vi "Example One Stage.vi"() -> ()   [LabVIEW 2019]
uses:
  Class/Controller/Controller.lvclass
  <vilib>/Platform/TimedLoop/XDataNode/timing_clust.ctl
  <vilib>/Platform/TimedLoop/XDataNode/nitl_modes.ctl
  <vilib>/Platform/TimedLoop/XDataNode/wakeup.ctl
  <vilib>/platform/TimedLoop/XDataNode/XDataNode.xnode
  <vilib>/Platform/TimedLoop/XDataNode/XDNodeRunTimeDep.lvlib
panel:
  out "Desired Position\n[selected units]":dbl
  out "Encoder position \n[selected units]":dbl
  in  "Tab Control":enum32{"Motion", "Settings"}(tab)
  in  "Zero Output":bool
  in  "Go to Home":bool
  in  "Scan Right":bool
  in  "Scan Left":bool
  in  "Continue":bool
  in  "Stop":bool
  in  "Make Step Right":bool
  in  "Step Size \n[selected units]":dbl=1.0 format="%#.2f"
  in  "Make Step Left":bool
  in  "Desired Speed \n[1µm/s or 0,01deg /s]":dbl=10000.0 format="%#.2f"
  in  "Desired Position \n[selected units]":dbl format="%#.2f"
  in  "Find Index":bool
  in  "Reset":bool
  out "error out":errorcluster
  in  "Working Units":string(combo)="1000000"
  out "StatusBits":T1
  out "Status Info":T2
  in  "Axis Resolution":string(combo)="312.5"
  in  "Axis Letter":string="X"
  in  "Baudrate":dbl=9600.0
  in  "COM Port":refnum<visa-resource-name>
  in  "Controller.lvclass":refnum<class "Controller.lvclass">
  out "Waveform Chart":dbl(graph)=-0.078
  in  "STOP PROGRAM":bool
  # "Visualization"
  # "Extra information"
  # "READ ME FIRST"
  # "Configuration"
  # "Stage 1"
  # "Driver 1"
  # "Stage 1"
  # "How to run:"
  # "BEFORE RUNNING:"
  # "1, Select COM Port"
  # "2. Select baudrate"
  # "3. For each axis:"
  # "3.1 Specify correct axis name (1 letter)"
  # "3.2 Specify correct resolution"
  # "4. Run VI"
  # "WHEN RUNNING, YOU HAVE TO FIRST PUSH \"FIND INDEX\" FOR EACH STAGE.\nThe stages will start moving and find its position. After that you can control the stages"
  # "NOTES: Do this only the first time"
  # "1. Replace the settings_default.txt file with\nthe file we provided on a USB stick."
  # "2.    Make sure there are no comments in the\nsettings_default.txt file. ONLY lines like: \"X:DPOS=100\" so NO \"%\" in front or at the end of the line."
  # "Position Information"
  # "STOP BUTTON"
  # "3.  In your settings_default.txt file:\nEvery line that contains SSPD or MSPD: multiply that value with:\n - 1000 for a lineair stage \n - 100 for a rotating stage"
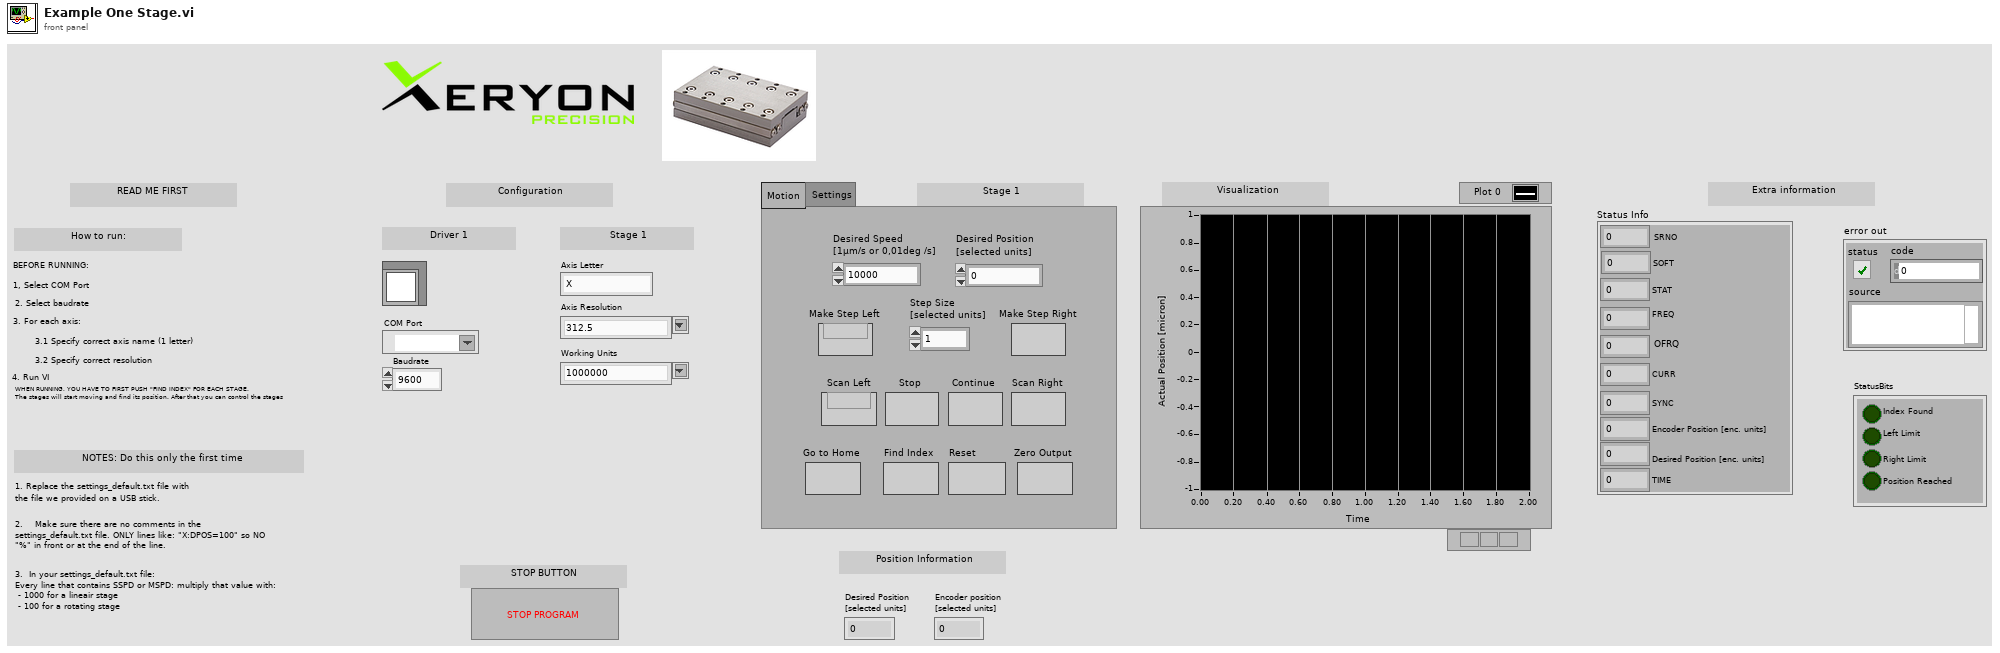
[diagram p1: front panel]
types:
  T1 = cluster{"Index Found":bool, "Left Limit":bool, "Right Limit":bool, "Position Reached":bool}
  T2 = cluster{"SRNO":dbl, "SOFT":dbl, "STAT":dbl, "FREQ":dbl, "OFRQ":dbl, "CURR":dbl, "SYNC":dbl, "Encoder Position [enc. units]":dbl, "Desired Position [enc. units]":dbl, "TIME":dbl}
  T3 = typedef "XDNodeRunTimeDep.lvlib/timing_clust.ctl" = cluster{"Expected End [f-1]":u64, "Actual End [f-1]":u64, "Finished Late? [f-1]":bool, "Expected End [i-1]":u64, "Actual End [i-1]":u64, "Finished Late? [i-1]":bool, "Expected Start [i]":u64, "Actual Start [i]":u64, "Expected Start [f]":u64, "Actual Start [f]":u64, "Source Name":string, "Structure Name":string, "Period":i64, "Deadline":i64, "Offset":i64, "Start":i64, "Priority":i32, "Timeout":i32, "Mode":T4, "Wakeup Reason":T5, "Error":errorcluster, "Source Type":string, "Secondary Source Type":string, "Global End Time":u64, "Global Start Time":u64, "Frame Duration":u64, "Iteration Duration":u64, "Assigned CPU":i32, "I/O Scan Engine Mode":u32}
  T4 = typedef "XDNodeRunTimeDep.lvlib/nitl_modes.ctl" = enum32{"No Change", "Process missed periods, maintain original phase", "Discard missed periods, maintain original phase", "Process missed periods, ignore original phase", "Discard missed periods, ignore original phase"}
  T5 = typedef "XDNodeRunTimeDep.lvlib/wakeup.ctl" = enum32{"Normal", "Aborted", "Asynchronous wakeup", "Timing source error", "Timed loop error", "Timeout"}
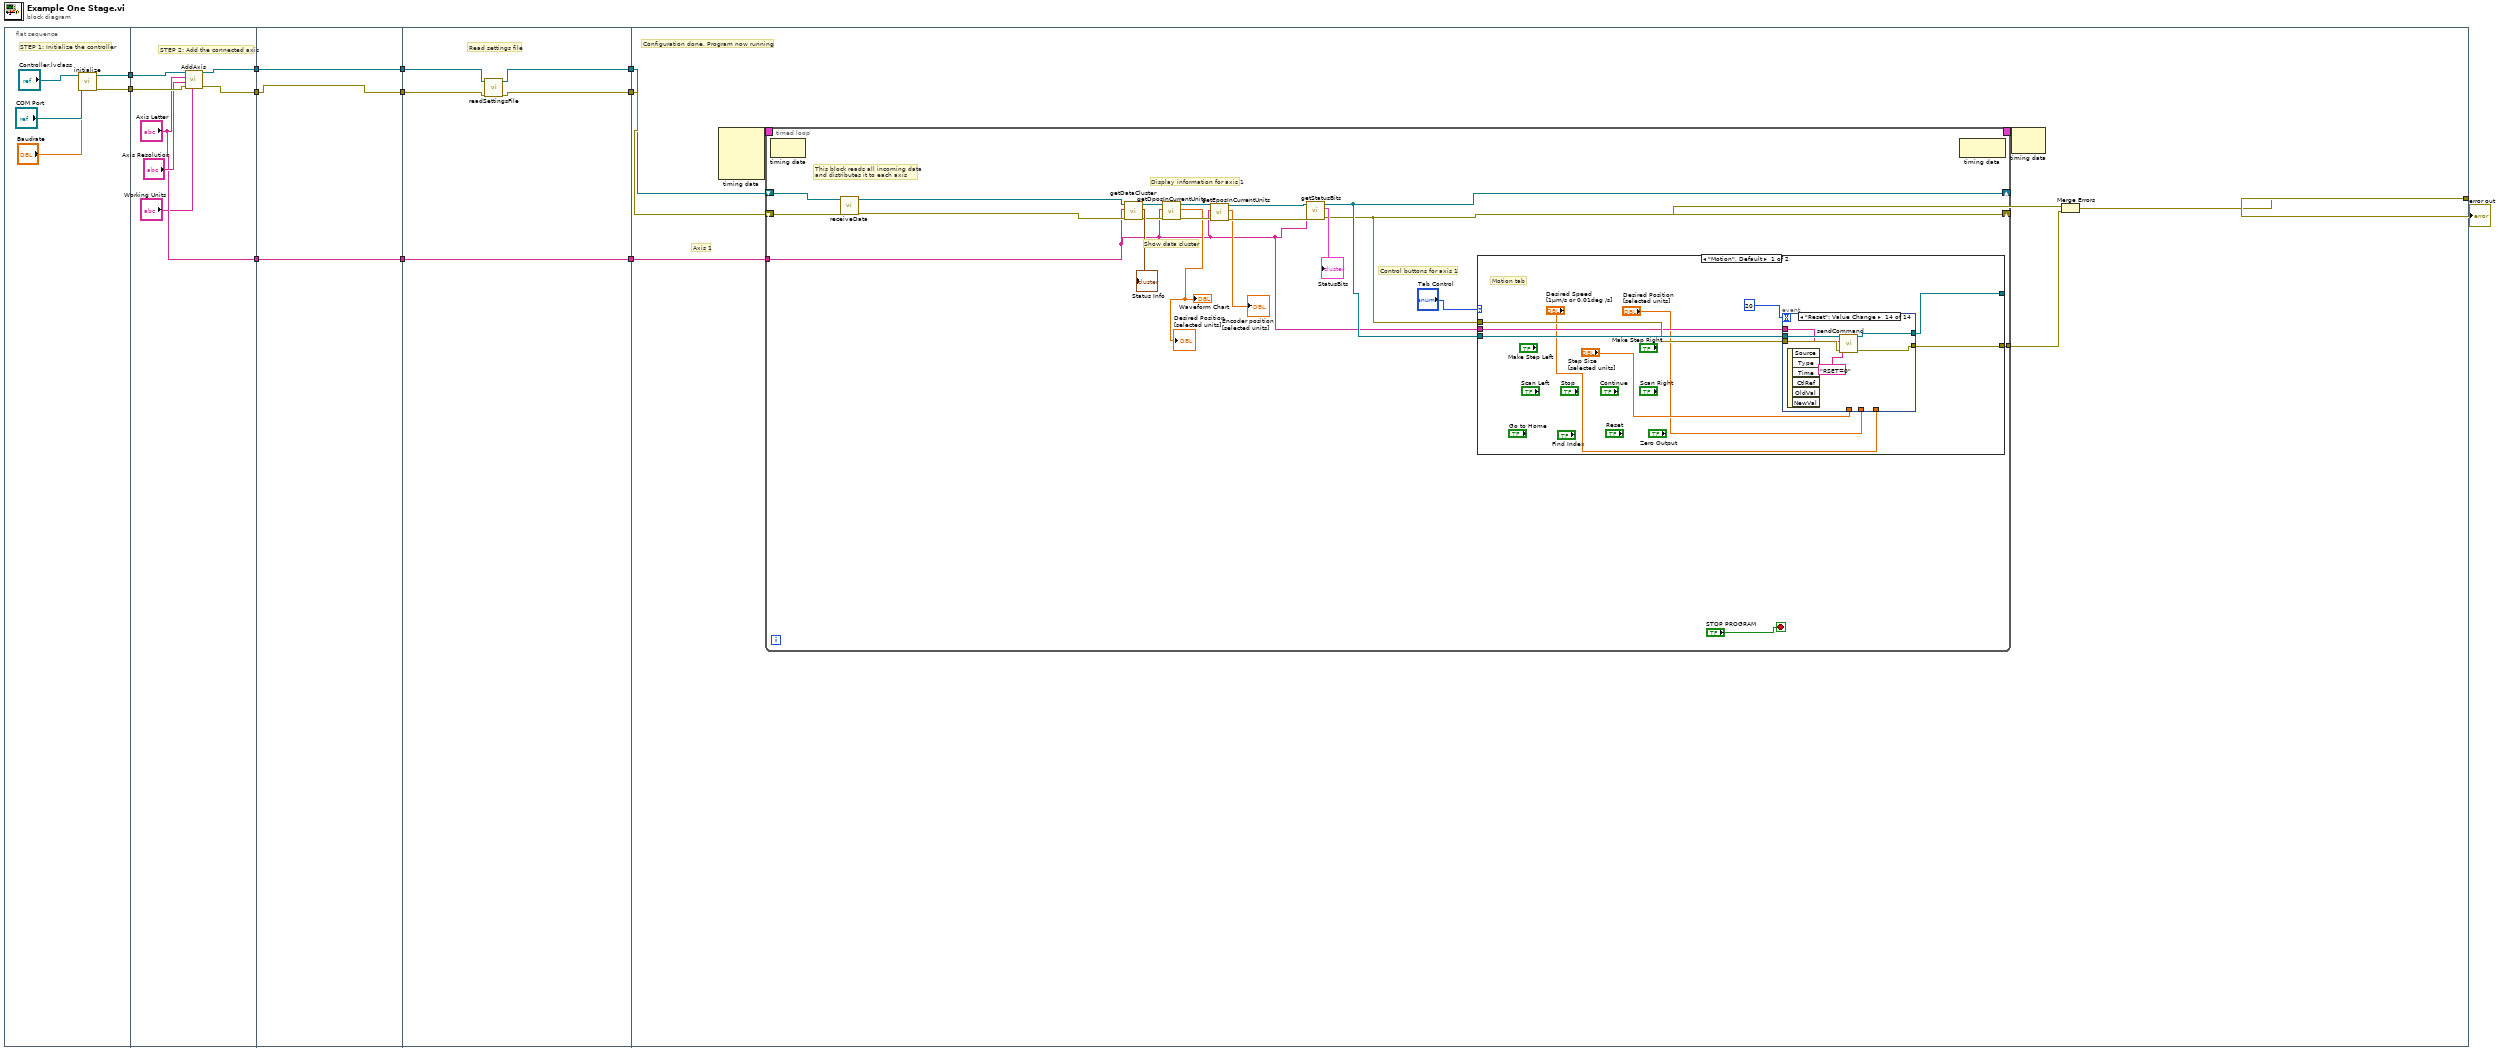
[diagram p0: block diagram]
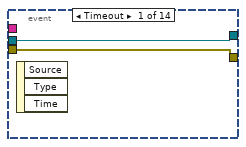
[diagram p2: hidden frame]
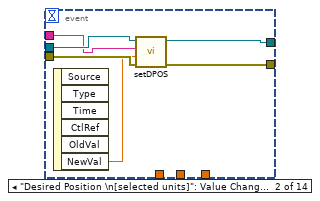
[diagram p3: hidden frame]
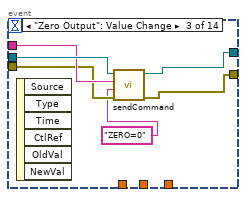
[diagram p4: hidden frame]
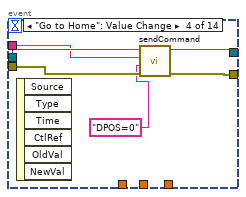
[diagram p5: hidden frame]
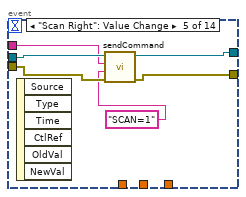
[diagram p6: hidden frame]
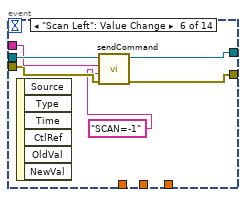
[diagram p7: hidden frame]
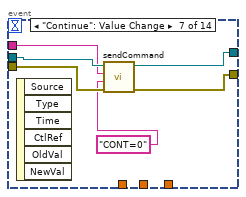
[diagram p8: hidden frame]
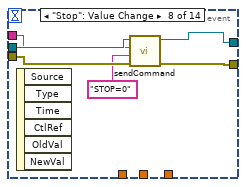
[diagram p9: hidden frame]
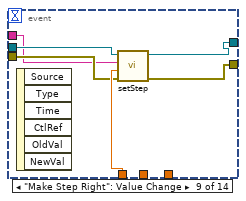
[diagram p10: hidden frame]
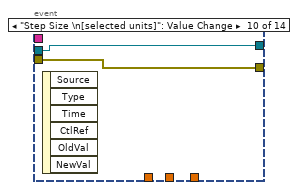
[diagram p11: hidden frame]
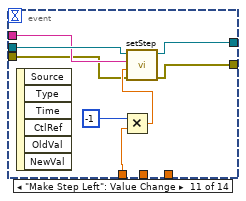
[diagram p12: hidden frame]
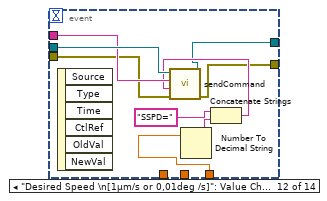
[diagram p13: hidden frame]
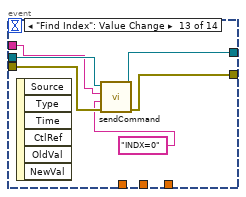
[diagram p14: hidden frame]
diagram:
  n1 = flat-sequence {
    tunnel: [w14] -> w12
    tunnel: [w13] -> w11
    tunnel: w12 -> [w24]
    tunnel: w11 -> [w23]
    tunnel: [w21] -> w10
    tunnel: [w20] -> w9
    tunnel: ["Axis Letter"] -> w8
    tunnel: w10 -> [w26]
    tunnel: w9 -> [w25]
    tunnel: [w27] -> w6
    tunnel: w8 -> [w27]
    tunnel: [w26] -> w4
    tunnel: [w25] -> w2
    tunnel: w6 -> [w32]
    tunnel: [w32] -> w5
    tunnel: w4 -> [w31]
    tunnel: [w29] -> w3
    tunnel: w2 -> [w30]
    tunnel: [w28] -> w1
    tunnel: w5 -> [w33]
    tunnel: w3 -> [w39]
    tunnel: w1 -> [w40]
    tunnel: [w35] -> w7
    frame #0 {
      # "STEP 1: Initialize the controller"
      n2 = call-dynamic "initialize.vi"("Baudrate"="Baudrate", "COM Port"="COM Port", "Controller in"="Controller.lvclass") -> ("error out"=w13:errorcluster, "Controller out"=w14:refnum<class "Controller.lvclass">)  [unwired: 7 in]
    }
    frame #1 {
      # "STEP 2: Add the connected axis"
      n3 = call-dynamic "AddAxis.vi"("Units"="Working Units", "error in (no error)"=w23, "Encoder Resolution"="Axis Resolution", "Axis Letter"="Axis Letter", "Controller in"=w24) -> ("error out"=w20:errorcluster, "Controller out"=w21:refnum<class "Controller.lvclass">)  [unwired: 5 in]
    }
    frame #2 {
    }
    frame #3 {
      # "Read settings file"
      n4 = call-dynamic "readSettingsFile.vi"("error in (no error)"=w30, "Controller in"=w31) -> ("error out"=w28:errorcluster, "Controller out"=w29:refnum<class "Controller.lvclass">)  [unwired: 8 in]
    }
    frame #4 {
      # "Axis 1"
      # "Configuration done. Program now running"
      n5 = node-c288() -> (w38:T3)  [unwired: 4 in]
      n6 = timed-loop {
        shift-right: [w44] -> _
        shift-left: w39 -> [w60]
        tunnel: w33 -> [w42]
        shift-right: [w43] -> w36
        shift-left: w40 -> [w47]
        timing: w38 -> [_]
        timing-out: [_] -> w37
        tunnel: [w41] -> w34
        stop <- "STOP PROGRAM" stop-if-true
        # "Control buttons for axis 1"
        # "Display information for axis 1"
        # "Show data cluster"
        # "This block reads all incoming data\nand distributes it to each axis"
        n7 = node-c288() -> ()  [unwired: 1 in, 1 out]
        n8 = call-dynamic "receiveData.vi"("error in (no error)"=w47, "Controller in"=w60) -> ("error out"=w58:errorcluster, "Controller out"=w59:refnum<class "Controller.lvclass">)  [unwired: 8 in]
        n9 = call-dynamic "getDataCluster.vi"("error in (no error)"=w58, "Axis Letter"=w42, "Controller in"=w59) -> ("error out"=w52:errorcluster, "Information"=→"Status Info":T2, "Controller out"=w55:refnum<class "Controller.lvclass">)  [unwired: 6 in]
        n10 = call-dynamic "getDposInCurrentUnits.vi"("error in (no error)"=w52, "Axis Letter"=w42, "Controller in"=w55) -> ("error out"=w51:errorcluster, "DPOS In Current Units"=→"Waveform Chart" →"Desired Position\n[selected units]":dbl, "Controller out"=w54:refnum<class "Controller.lvclass">)  [unwired: 6 in]
        n11 = call-dynamic "getEposInCurrentUnits.vi"("error in (no error)"=w51, "Axis Letter"=w42, "Controller in"=w54) -> ("error out"=w50:errorcluster, "EPOS In Current Units"=→"Encoder position \n[selected units]":dbl, "Controller out"=w53:refnum<class "Controller.lvclass">)  [unwired: 6 in]
        n12 = call-dynamic "getStatusBits.vi"("error in (no error)"=w50, "Axis Letter"=w42, "Controller in"=w53) -> ("error out"=w43:errorcluster, "StatusBits"=→"StatusBits":T1, "Controller out"=w44:refnum<class "Controller.lvclass">)  [unwired: 6 in]
        n13 = case shown="\"Motion\", Default" "Tab Control" {
          tunnel: w44 -> [w69 w151]
          tunnel: w43 -> [w68 w152]
          tunnel: [w67 w151] -> _
          tunnel: [w66 w152] -> w41
          tunnel: w42 -> [w64 _]
          frame "Motion", Default {
            # "Motion tab"
            n14 = event shown="[13] \"Reset\": Value Change" {
              selector: _ -> [_ _ _ _ _ _ _ _ _ _ _ _ _ _]
              dyn-events: _ -> [_ _ _ _ _ _ _ _ _ _ _ _ _ _]
              timeout: 20 -> [_ _ _ _ _ _ _ _ _ _ _ _ _ _]
              tunnel: w69 -> [w71 w77 w83 w89 w95 w101 w107 w113 w117 w121 w127 w138 w144 w150]
              tunnel: w68 -> [w70 w76 w81 w87 w93 w99 w105 w111 w118 w120 w124 w136 w142 w149]
              tunnel: [w71 w74 w79 w84 w91 w97 w103 w109 w115 w121 w122 w130 w140 w146] -> w67
              tunnel: [w70 w75 w80 w86 w92 w98 w104 w110 w114 w120 w123 w131 w141 w145] -> w66
              tunnel: w64 -> [_ w72 w82 w88 w94 w100 w106 w112 w116 _ w126 w137 w143 w148]
              tunnel: "Step Size \n[selected units]" -> [_ _ _ _ _ _ _ _ w119 _ w128 _ _ _]
              tunnel: "Desired Position \n[selected units]" -> [_ _ _ _ _ _ _ _ _ _ _ _ _ _]
              tunnel: "Desired Speed \n[1µm/s or 0,01deg /s]" -> [_ _ _ _ _ _ _ _ _ _ _ w135 _ _]
              event Timeout {
                n15 = event-data() -> ()  [unwired: 1 in, 3 out]
              }
              event "Desired Position \n[selected units]": Value Change {
                n16 = event-data() -> ("NewVal"=w73:dbl)  [unwired: 1 in, 5 out]
                n17 = call-dynamic "setDPOS.vi"("error in (no error)"=w76, "DPOS In Current Units"=w73, "Axis Letter"=w72, "Controller in"=w77) -> ("error out"=w75:errorcluster, "Controller out"=w74:refnum<class "Controller.lvclass">)  [unwired: 6 in]
              }
              event "Zero Output": Value Change {
                n18 = event-data() -> ()  [unwired: 1 in, 6 out]
                n19 = call-dynamic "sendCommand.vi"("error in (no error)"=w81, "Command"="ZERO=0", "Axis Letter"=w82, "Controller in"=w83) -> ("error out"=w80:errorcluster, "Controller out"=w79:refnum<class "Controller.lvclass">)  [unwired: 6 in]
              }
              event "Go to Home": Value Change {
                n20 = event-data() -> ()  [unwired: 1 in, 6 out]
                n21 = call-dynamic "sendCommand.vi"("error in (no error)"=w87, "Command"="DPOS=0", "Axis Letter"=w88, "Controller in"=w89) -> ("error out"=w86:errorcluster, "Controller out"=w84:refnum<class "Controller.lvclass">)  [unwired: 6 in]
              }
              event "Scan Right": Value Change {
                n22 = event-data() -> ()  [unwired: 1 in, 6 out]
                n23 = call-dynamic "sendCommand.vi"("error in (no error)"=w93, "Command"="SCAN=1", "Axis Letter"=w94, "Controller in"=w95) -> ("error out"=w92:errorcluster, "Controller out"=w91:refnum<class "Controller.lvclass">)  [unwired: 6 in]
              }
              event "Scan Left": Value Change {
                n24 = event-data() -> ()  [unwired: 1 in, 6 out]
                n25 = call-dynamic "sendCommand.vi"("error in (no error)"=w99, "Command"="SCAN=-1", "Axis Letter"=w100, "Controller in"=w101) -> ("error out"=w98:errorcluster, "Controller out"=w97:refnum<class "Controller.lvclass">)  [unwired: 6 in]
              }
              event "Continue": Value Change {
                n26 = event-data() -> ()  [unwired: 1 in, 6 out]
                n27 = call-dynamic "sendCommand.vi"("error in (no error)"=w105, "Command"="CONT=0", "Axis Letter"=w106, "Controller in"=w107) -> ("error out"=w104:errorcluster, "Controller out"=w103:refnum<class "Controller.lvclass">)  [unwired: 6 in]
              }
              event "Stop": Value Change {
                n28 = event-data() -> ()  [unwired: 1 in, 6 out]
                n29 = call-dynamic "sendCommand.vi"("error in (no error)"=w111, "Command"="STOP=0", "Axis Letter"=w112, "Controller in"=w113) -> ("error out"=w110:errorcluster, "Controller out"=w109:refnum<class "Controller.lvclass">)  [unwired: 6 in]
              }
              event "Make Step Right": Value Change {
                n30 = event-data() -> ()  [unwired: 1 in, 6 out]
                n31 = call-dynamic "setStep.vi"("error in (no error)"=w118, "Step Value"=w119, "Axis Letter"=w116, "Controller in"=w117) -> ("error out"=w114:errorcluster, "Controller out"=w115:refnum<class "Controller.lvclass">)  [unwired: 6 in]
              }
              event "Step Size \n[selected units]": Value Change {
                n32 = event-data() -> ()  [unwired: 1 in, 6 out]
              }
              event "Make Step Left": Value Change {
                n33 = event-data() -> ()  [unwired: 1 in, 6 out]
                n34 = Multiply(x=-1, y=w128) -> (x*y=w125:dbl)
                n35 = call-dynamic "setStep.vi"("error in (no error)"=w124, "Step Value"=w125, "Axis Letter"=w126, "Controller in"=w127) -> ("error out"=w123:errorcluster, "Controller out"=w122:refnum<class "Controller.lvclass">)  [unwired: 6 in]
              }
              event "Desired Speed \n[1µm/s or 0,01deg /s]": Value Change {
                n36 = event-data() -> ()  [unwired: 1 in, 6 out]
                n37 = Number To Decimal String(number=w135) -> (decimal integer string=w133:string)  [unwired: 1 in]
                n38 = Concatenate Strings("SSPD=", w133) -> (w132:string)
                n39 = call-dynamic "sendCommand.vi"("error in (no error)"=w136, "Command"=w132, "Axis Letter"=w137, "Controller in"=w138) -> ("error out"=w131:errorcluster, "Controller out"=w130:refnum<class "Controller.lvclass">)  [unwired: 6 in]
              }
              event "Find Index": Value Change {
                n40 = event-data() -> ()  [unwired: 1 in, 6 out]
                n41 = call-dynamic "sendCommand.vi"("error in (no error)"=w142, "Command"="INDX=0", "Axis Letter"=w143, "Controller in"=w144) -> ("error out"=w141:errorcluster, "Controller out"=w140:refnum<class "Controller.lvclass">)  [unwired: 6 in]
              }
              event "Reset": Value Change {
                n42 = event-data() -> ()  [unwired: 1 in, 6 out]
                n43 = call-dynamic "sendCommand.vi"("error in (no error)"=w149, "Command"="RSET=0", "Axis Letter"=w148, "Controller in"=w150) -> ("error out"=w145:errorcluster, "Controller out"=w146:refnum<class "Controller.lvclass">)  [unwired: 6 in]
              }
            }
          }
          frame "Settings" {
          }
        }
        n44 = node-c288() -> ()  [unwired: 1 in, 1 out]
      }
      n45 = node-c288(w37) -> ()  [unwired: 1 out]
      n46 = Merge Errors(w36, w34) -> (w35:errorcluster)
    }
  }
  "error out" <- w7
